vi "GetCode.vi"(9 "Error in":errorcluster) -> (1 "Code":i32)   [LabVIEW 2017, in "GPError.lvlib"]
doc: "Returns <B>Code</B> from <B>Error in</B>. For appended errors the code from the primary error/warning is returned only.\n\nThis VI is inlined.\n\nSteen Schmidt\nGPower\n17/7 2013"
uses:
  GPError.lvlib
panel:
  # "Copyright © 2013\nSteen Schmidt, GPower\nSee enclosed license file for terms and conditions"
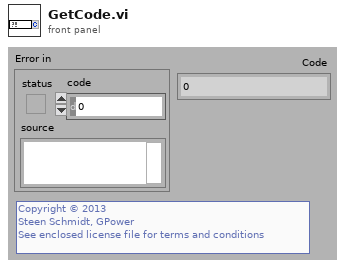
[diagram p1: front panel]
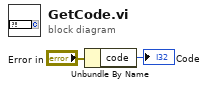
[diagram p0: block diagram]
diagram:
  n1 = Unbundle By Name("Error in") -> ("code"=→"Code":i32)
